vi "DecToHex.vi"(2 "Decimal . Decimal Representation":dbl=2.545 format="%.4f") -> (0 "HEX . HEX representation":string="2.8B851")   [LabVIEW 2022 SP3]
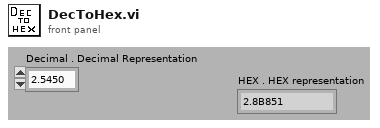
[diagram p1: front panel]
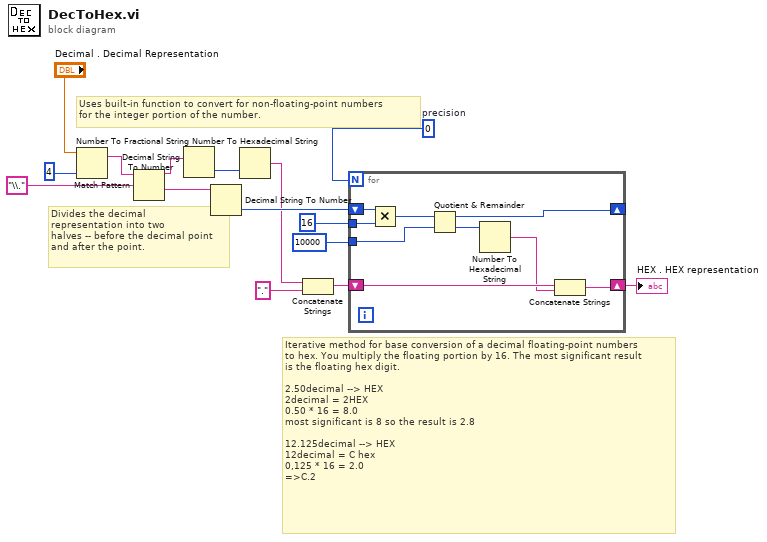
[diagram p0: block diagram]
diagram:
  w1 = 0  # precision
  # "Iterative method for base conversion of a decimal floating-point numbers \nto hex. You multiply the floating portion by 16. The most significant result\nis the floating hex digit.\n\n2.50decimal --> HEX\n2decimal = 2HEX\n0.50 * 16 = 8.0\nmost significant is 8 so the result is 2.8\n\n12.125decimal --> HEX\n12decimal = C hex\n0,125 * 16 = 2.0\n=>C.2"
  # "Uses built-in function to convert for non-floating-point numbers\nfor the integer portion of the number."
  # "Divides the decimal\nrepresentation into two\nhalves -- before the decimal point\nand after the point."
  n1 = Number To Fractional String(number="Decimal . Decimal Representation", precision (6)=i16 4) -> (F-format string=w14:string)  [unwired: 2 out]
  n2 = Match Pattern(string=w14, regular expression="\\.") -> (before substring=w12:string, after substring=w11:string)  [unwired: 3 out]
  n3 = Decimal String To Number(string=w12) -> (number=w10:i32)  [unwired: 3 out]
  n4 = Decimal String To Number(string=w11) -> (number=w9:i32)  [unwired: 3 out]
  n5 = Number To Hexadecimal String(2:w10) -> (0:w4:string)  [unwired: 1 out]
  n6 = Concatenate Strings(w4, "." ("Substring")) -> (w5:string)
  n7 = for {
    N: w1 -> [_]
    shift-right: [w20] -> _
    shift-left: w9 -> [w23]
    tunnel: 16 ("y") -> [w22]
    tunnel: 10000 ("y") -> [w21]
    shift-right: [w17] -> w6
    shift-left: w5 -> [w18]
    n8 = Multiply(x=w23, y=w22) -> (x*y=w24:i32)
    n9 = Quotient & Remainder(x=w24, y=w21) -> (x-y*floor(x/y)=w20:i32, floor(x/y)=w19:i32)
    n10 = Number To Hexadecimal String(2:w19) -> (0:w16:string)  [unwired: 1 out]
    n11 = Concatenate Strings(w18, w16) -> (w17:string)
  }
  "HEX . HEX representation" <- w6
